vi "add modification.vi"(8 "error in":errorcluster, 10 "VI modification":refnum<class "VI modification.lvclass">, 11 "vi modification tool in":refnum<class "VI modification collection.lvclass">) -> (0 "error out":errorcluster, 3 "vi modification tool out":refnum<class "VI modification collection.lvclass">)   [LabVIEW 2013, in "VI modification collection.lvclass"]
uses:
  VI modification collection.lvclass
  VI modification.lvclass
  VI modification collection.lvclass/VI modification collection.ctl
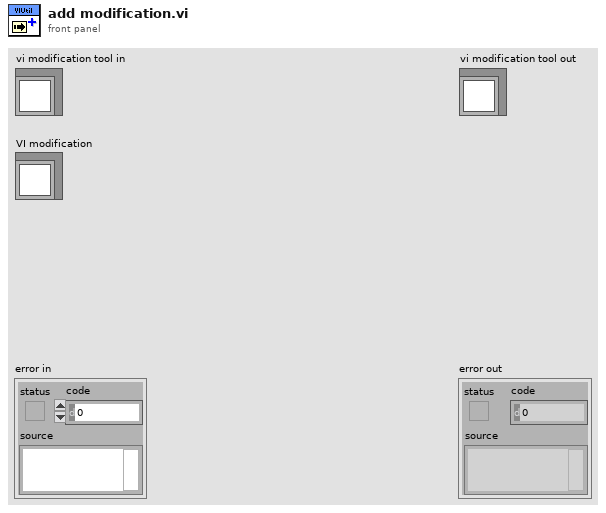
[diagram p1: front panel]
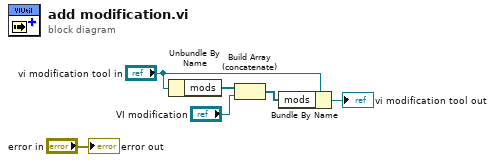
[diagram p0: block diagram]
diagram:
  n1 = Unbundle By Name("vi modification tool in") -> ("mods"=w6:refnum<class "VI modification.lvclass">[])
  n2 = Build Array (concatenate)(w6, "VI modification") -> (w2:refnum<class "VI modification.lvclass">[])
  n3 = Bundle By Name(cluster="vi modification tool in", "mods"=w2) -> (→"vi modification tool out":refnum<class "VI modification collection.lvclass">)
  "error out" <- "error in"
